vi "NI-DP__ReceiveData.vi"(6 "timeout [ms]":u32, 8 "error in":errorcluster, 11 "UDP Network Connection in":refnum<k16>) -> (0 "error out":errorcluster, 1 "param 2":string, 2 "param 1":string, 3 "UDP Network Connection out":refnum<k16>, 4 "UDP-NI Message":T1 {"Command" items=["0x01: Get Type & Hostname"=1, "0x03: Set IP 1"=3, "0x04: Set IP 2"=4, "0x08: Acknowledge"=8, "0x0A: Reboot"=10, "0x20: ???"=32, "0x21: ???"=33, "0xF2: System State"=242, "0xF4: System Details"=244]}, 5 "IP (MAC)":string)   [LabVIEW 2014, in "hse-network.lvlib"]
doc: "____\nHAMPEL SOFTWARE ENGINEERING v0.7.0 (2018-07-16 18:12)"
uses:
  hse-network.lvlib
  NI-DP__MessageStructure.ctl
  NI-DP__Commands.ctl
  hse-misc/hse-misc.lvlib
panel:
  out "length":i32
  out "UDP RX Data (Hex)":string
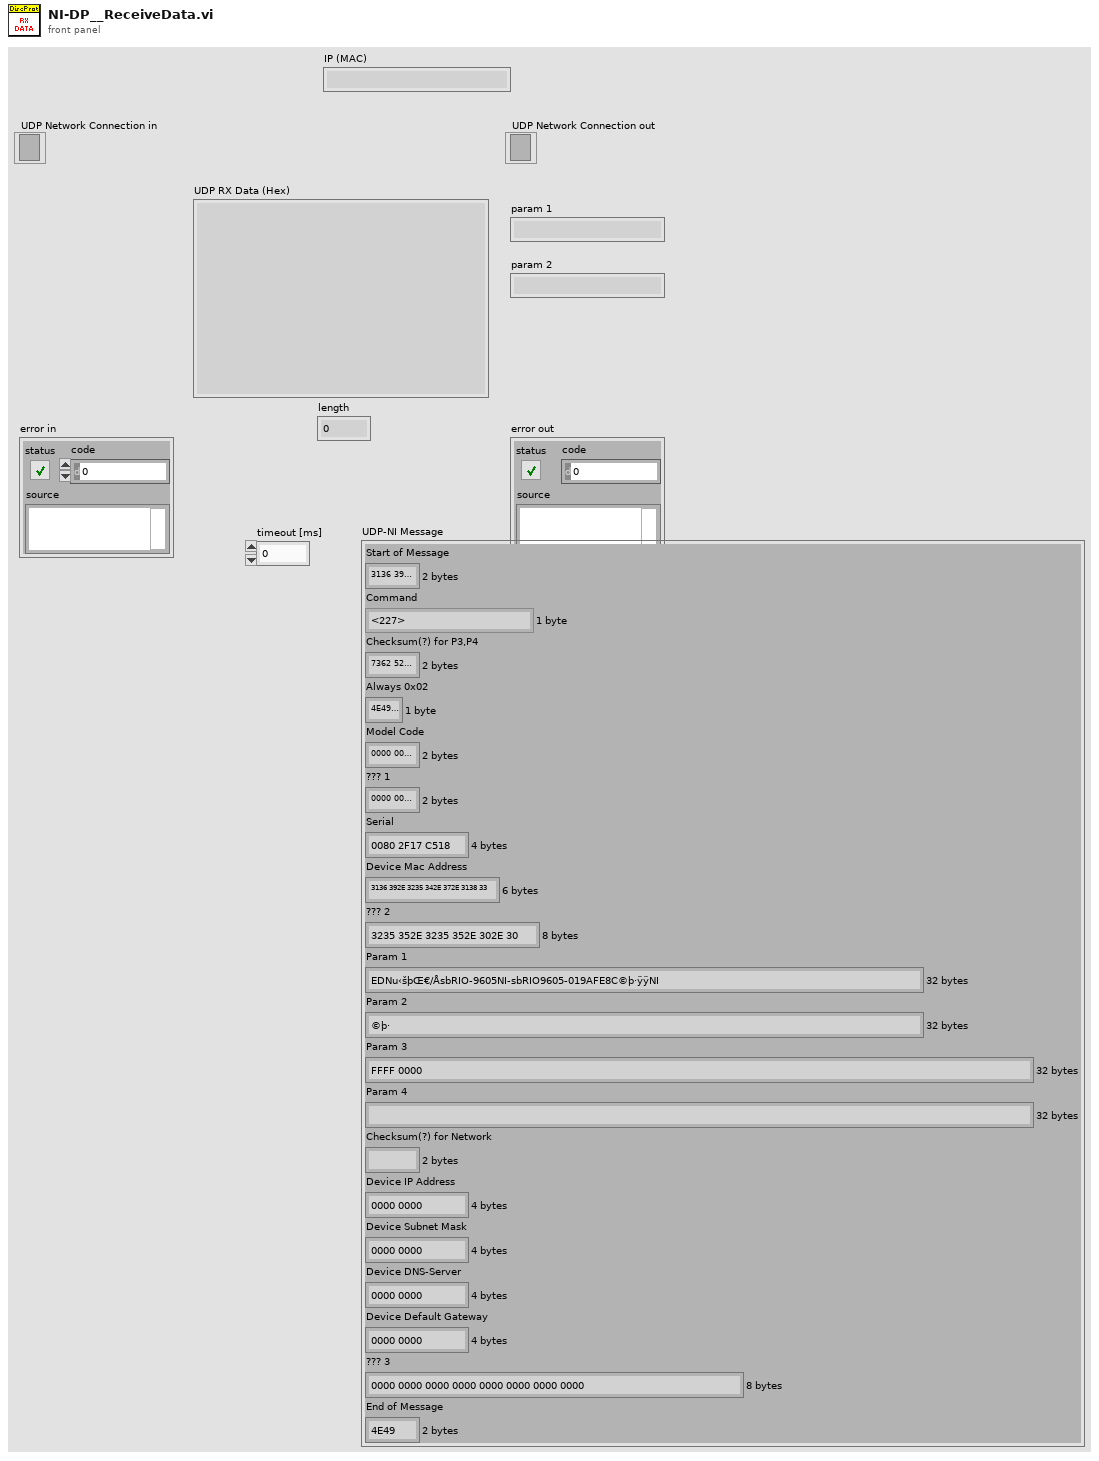
[diagram p1: front panel]
types:
  T1 = typedef "hse-network.lvlib/NI-DP__MessageStructure.ctl" = cluster{"Start of Message":string, "Command":T2, "Checksum(?) for P3,P4":string, "Always 0x02":string, "Model Code":string, "??? 1":string, "Serial":string, "Device Mac Address":string, "??? 2":string, "Param 1":string, "Param 2":string, "Param 3":string, "Param 4":string, "Checksum(?) for Network":string, "Device IP Address":string, "Device Subnet Mask":string, "Device DNS-Server":string, "Device Default Gateway":string, "??? 3":string, "End of Message":string}
  T2 = typedef "hse-network.lvlib/NI-DP__Commands.ctl" = u8
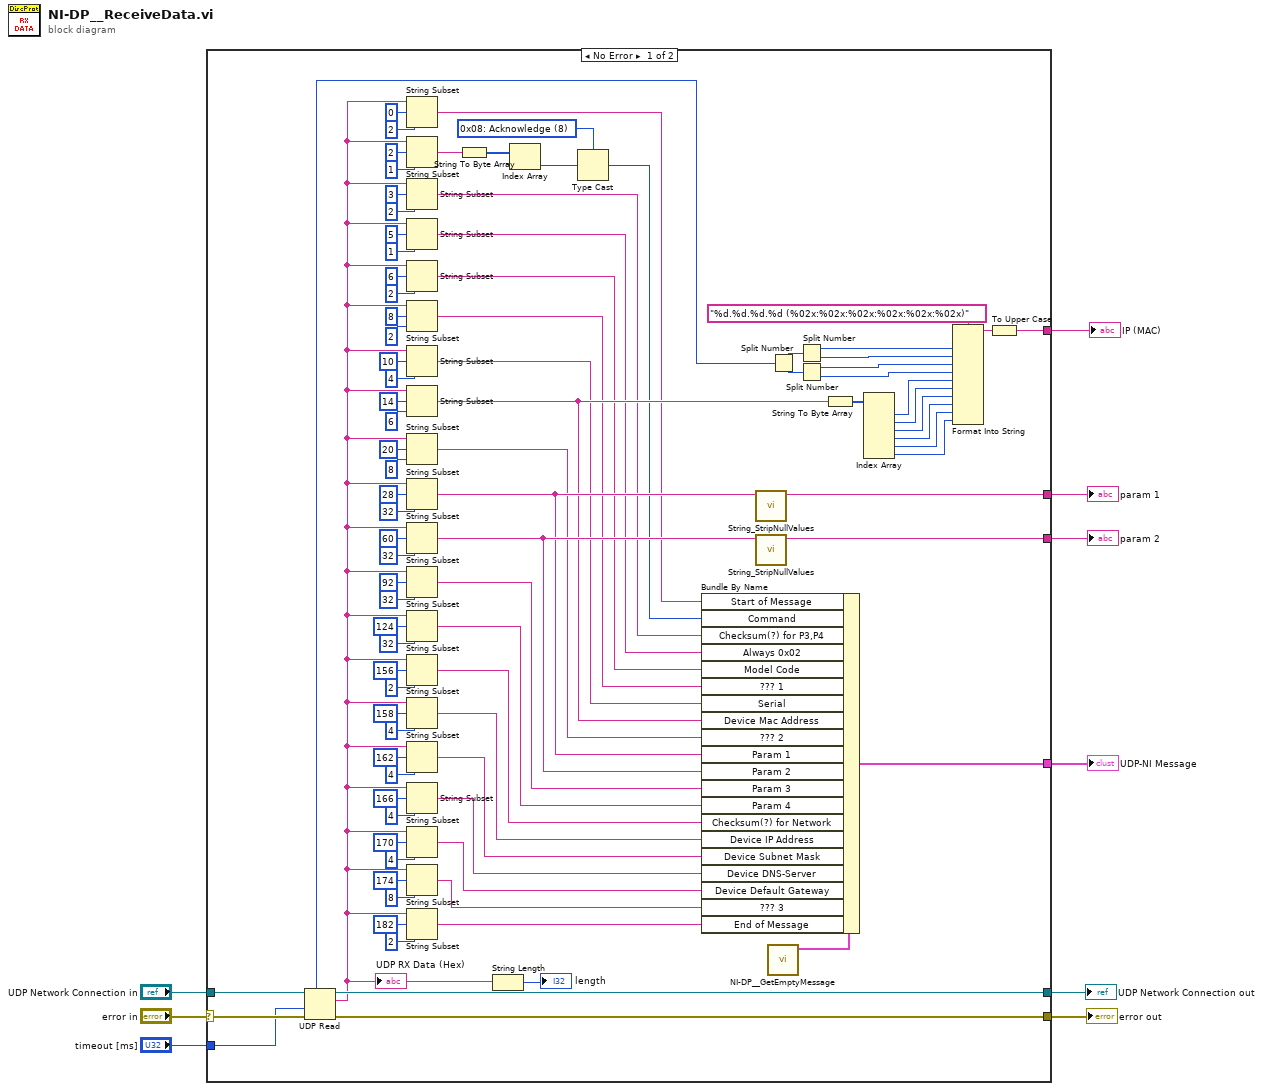
[diagram p0: block diagram]
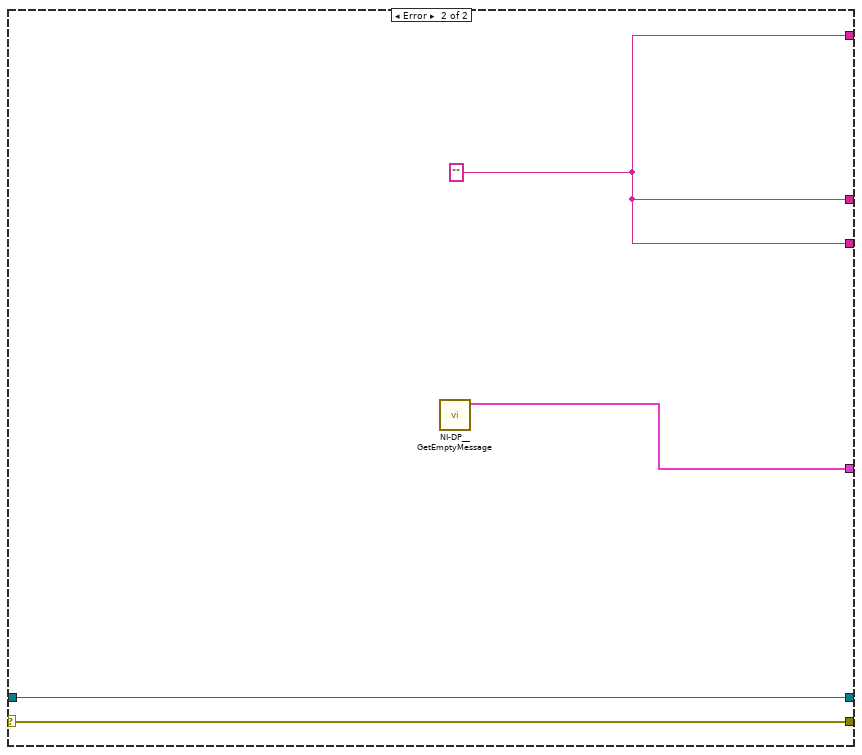
[diagram p2: hidden frame]
diagram:
  n1 = case shown="No Error" "error in" {
    selector: "error in" -> [w88 w105]
    tunnel: [w101 w104] -> w9
    tunnel: "UDP Network Connection in" -> [w100 w104]
    tunnel: [w92 w105] -> w7
    tunnel: [w64 w103] -> w6
    tunnel: [w10 w103] -> w5
    tunnel: [w11 w103] -> w4
    tunnel: "timeout [ms]" -> [w87 _]
    tunnel: [w65 w102] -> w1
    frame No Error {
      w21 = T2 8 items=["0x01: Get Type & Hostname"=1, "0x03: Set IP 1"=3, "0x04: Set IP 2"=4, "0x08: Acknowledge"=8, "0x0A: Reboot"=10, "0x20: ???"=32, "0x21: ???"=33, "0xF2: System State"=242, "0xF4: System Details"=244] ("Command")
      n2 = UDP Read(connection ID=w100, timeout ms (25000)=w87, 8:w88) -> (data out=w15:string, error out=w92:errorcluster, 3:w101:refnum<k16>, 6:w25:u32)  [unwired: 1 in, 1 out]
      "UDP RX Data (Hex)" <- w15
      n3 = String Subset(string=w15, offset (0)=0, length (rest)=2 ("length (rest)")) -> (substring=w29:string)
      n4 = String Subset(string=w15, offset (0)=2, length (rest)=1 ("length (rest)")) -> (substring=w24:string)
      n5 = String Subset(string=w15, offset (0)=3, length (rest)=2 ("length (rest)")) -> (substring=w28:string)
      n6 = String Subset(string=w15, offset (0)=5, length (rest)=1 ("length (rest)")) -> (substring=w27:string)
      n7 = String Subset(string=w15, offset (0)=6, length (rest)=2 ("length (rest)")) -> (substring=w26:string)
      n8 = String Subset(string=w15, offset (0)=8, length (rest)=2 ("length (rest)")) -> (substring=w30:string)
      n9 = String Subset(string=w15, offset (0)=10, length (rest)=4 ("length (rest)")) -> (substring=w39:string)
      n10 = String Subset(string=w15, offset (0)=14, length (rest)=6 ("length (rest)")) -> (substring=w40:string)
      n11 = String Subset(string=w15, offset (0)=20, length (rest)=8 ("length (rest)")) -> (substring=w41:string)
      n12 = String Subset(string=w15, offset (0)=28, length (rest)=32 ("length (rest)")) -> (substring=w44:string)
      n13 = String Subset(string=w15, offset (0)=60, length (rest)=32 ("length (rest)")) -> (substring=w45:string)
      n14 = String Subset(string=w15, offset (0)=92, length (rest)=32 ("length (rest)")) -> (substring=w46:string)
      n15 = String Subset(string=w15, offset (0)=124, length (rest)=32 ("length (rest)")) -> (substring=w47:string)
      n16 = String Subset(string=w15, offset (0)=156, length (rest)=2 ("length (rest)")) -> (substring=w48:string)
      n17 = String Subset(string=w15, offset (0)=158, length (rest)=4 ("length (rest)")) -> (substring=w51:string)
      n18 = String Subset(string=w15, offset (0)=162, length (rest)=4 ("length (rest)")) -> (substring=w52:string)
      n19 = String Subset(string=w15, offset (0)=166, length (rest)=4 ("length (rest)")) -> (substring=w53:string)
      n20 = String Subset(string=w15, offset (0)=170, length (rest)=4 ("length (rest)")) -> (substring=w12:string)
      n21 = String Subset(string=w15, offset (0)=174, length (rest)=8 ("length (rest)")) -> (substring=w13:string)
      n22 = String Subset(string=w15, offset (0)=182, length (rest)=2 ("length (rest)")) -> (substring=w14:string)
      n23 = String To Byte Array(string=w24) -> (unsigned byte array=w23:u8[])
      n24 = String Length(string=w15) -> (length=→"length":i32)
      n25 = Index Array(array=w23) -> (element=w22:u8)  [unwired: 1 in]
      n26 = Type Cast(type=w21, x=w22) -> (*(type *) &x=w20:T2)
      n27 = call "String_StripNullValues.vi"("str in"=w44) -> ("str (stripped)"=w11:string)  [unwired: 10 in]
      n28 = call "String_StripNullValues.vi"("str in"=w45) -> ("str (stripped)"=w10:string)  [unwired: 10 in]
      n29 = call "NI-DP__GetEmptyMessage.vi"() -> ("NI-DP__EmptyMessage"=w66:T1)  [unwired: 11 in]
      n30 = Bundle By Name(cluster=w66, "Start of Message"=w29, "Command"=w20, "Checksum(?) for P3,P4"=w28, "Always 0x02"=w27, "Model Code"=w26, "??? 1"=w30, "Serial"=w39, "Device Mac Address"=w40, "??? 2"=w41, "Param 1"=w44, "Param 2"=w45, "Param 3"=w46, "Param 4"=w47, "Checksum(?) for Network"=w48, "Device IP Address"=w51, "Device Subnet Mask"=w52, "Device DNS-Server"=w53, "Device Default Gateway"=w12, "??? 3"=w13, "End of Message"=w14) -> (w65:T1)
      n31 = Split Number(x=w25) -> (hi(x)=w99:u16, lo(x)=w98:u16)
      n32 = Split Number(x=w99) -> (hi(x)=w96:u8, lo(x)=w95:u8)
      n33 = Split Number(x=w98) -> (hi(x)=w94:u8, lo(x)=w93:u8)
      n34 = String To Byte Array(string=w40) -> (unsigned byte array=w86:u8[])
      n35 = Index Array(array=w86) -> (element #1=w85:u8, element #2=w84:u8, element #3=w83:u8, element #4=w82:u8, element #5=w81:u8, element #6=w80:u8)  [unwired: 6 in]
      n36 = Format Into String(format string="%d.%d.%d.%d (%02x:%02x:%02x:%02x:%02x:%02x)", w96, w95, w94, w93, w85, w84, w83, w82, w81, w80) -> (resulting string=w79:string)  [unwired: 2 in, 1 out]
      n37 = To Upper Case(1:w79) -> (0:w64:string)
    }
    frame Error {
      w103 = "" ("result string")
      n38 = call "NI-DP__GetEmptyMessage.vi"() -> ("NI-DP__EmptyMessage"=w102:T1)  [unwired: 11 in]
    }
  }
  "UDP Network Connection out" <- w9
  "error out" <- w7
  "IP (MAC)" <- w6
  "param 2" <- w5
  "param 1" <- w4
  "UDP-NI Message" <- w1
